vi "PI_GCS2_All_VIs.vi"   [LabVIEW 2020]
doc: "This VI contains all high level and low level VIs valid for PI GCS2 devices. \nSee diagram for a survey of all PI GCS2 high level and low level VIs. \nMenu / Browse / Show VI Hierarchy will show the file paths of the VIs. \nGlobal Variables are shown as Control as well as Indicator."
uses:
  Low Level/Communication.llb/Global1.vi
  Low Level/General command.llb/Controller names.ctl
  Low Level/Support.llb/Unbunde/bundle interface clusters for PI Terminal.vi
  Low Level/Communication.llb/Available DLL interfaces.ctl
  Low Level/Communication.llb/Available DLLs.ctl
  Low Level/Communication.llb/Available interfaces.ctl
  Low Level/Communication.llb/Termination character.ctl
  Low Level/General command.llb/Global2 (Array).vi
  Low Level/Communication.llb/Global DaisyChain.vi
  Low Level/Support.llb/HasCommandArray_Query.vi
  Low Level/Support.llb/GCSArray_regex_selector.ctl
  Low Level/Communication.llb/Syntax.ctl
  Low Level/General command.llb/CommandInfo.ctl
  Low Level/General command.llb/MemoryType.ctl
  Low Level/General command.llb/Parameter Set.ctl
  Low Level/General command.llb/ParameterInfoSet.ctl
  Low Level/General command.llb/UnitDescription.ctl
  Low Level/Special command.llb/UserCommandLevel.ctl
  Low Level/Communication.llb/Configuration Setup State.ctl
  Low Level/General command.llb/HardwareInfo.ctl
  Low Level/General command.llb/DynamicHardwareInfo.ctl
  Low Level/General command.llb/FirmwareInfo.ctl
  Low Level/Special command.llb/RecorderStatus.ctl
  Low Level/Special command.llb/RecorderTraceConfiguration.ctl
  Low Level/Special command.llb/RecorderTriggerConfiguration.ctl
  Low Level/Special command.llb/DriveStateMachine.ctl
  Low Level/Special command.llb/ModeOfOperation.ctl
  Low Level/General command.llb/AxisStatus.ctl
  Low Level/General command.llb/SystemStatus.ctl
  Low Level/General command.llb/Status.ctl
panel:
  # "PI GCS2 LabVIEW driver set"
  # "This VI contains all high level and low level VIs valid for PI GCS2 devices. See diagram for a survey of all PI GCS2 high level and low level VIs. Menu / Browse / Show VI Hierarchy will show the file paths of the VIs. Global Variables are shown as Control as well as Indicator."
types:
  T1 = typedef "Status.ctl" = cluster{"Element":string, "Status bits":bool[]}
  T2 = typedef "SystemStatus.ctl" = cluster{"Element":string, "Command Error":bool, "Critical Error":bool, "Information":bool, "Warning":bool}
  T3 = typedef "AxisStatus.ctl" = cluster{"Element":string, "Error":bool, "EAX?":bool, "Drive State Machine":T4, "Mode of Operation":T5, "OL/CL control active?":bool, "ONT?":bool, "In Motion":bool, "FRF?":bool, "IPR":bool, "Plim":bool, "Nlim":bool}
  T4 = typedef "DriveStateMachine.ctl" = u16
  T5 = typedef "ModeOfOperation.ctl" = enum16{"Open", "Open-Loop Position", "Closed-Loop Position", "Open-Loop Velocity", "Closed-Loop Velocity", "Open-Loop Force", "Closed-Loop Force", "Step Operation"}
  T6 = typedef "RecorderTriggerConfiguration.ctl" = cluster{"RecorderID":string, "RecorderTrigger":string, "AxisID":string, "Recurring":string}
  T7 = typedef "RecorderTraceConfiguration.ctl" = cluster{"RecorderID":string, "TraceID":i32, "Container Unit":string, "Function Unit":string, "ParameterID":i32}
  T8 = typedef "RecorderStatus.ctl" = enum16{"RUN", "CFG", "WAIT"}
  T9 = typedef "FirmwareInfo.ctl" = cluster{"Container Unit":string, "Function Unit":string, "ID":string, "Mathccode":string, "Version":string, "Date":string, "Compatibility":string, "Description":string}
  T10 = typedef "DynamicHardwareInfo.ctl" = cluster{"Property":string, "Type":string, "Value":string}
  T11 = typedef "HardwareInfo.ctl" = cluster{"Matchcode":string, "Version":string, "Serial Number":string, "Date":string, "Dynamic Hardware":cluster{"Property":string, "Type":string, "Value":string}[], "Firmware":cluster{"Container Unit":string, "Function Unit":string, "ID":string, "Mathccode":string, "Version":string, "Date":string, "Compatibility":string, "Description":string}[]}
  T12 = typedef "Configuration Setup State.ctl" = enum16{"Do nothing", "Initialize indicators", "Select Connection", "TCP/IP Connection", "RS232 Connection", "USB Connection", "Board Connection", "DaisyChain Connection", "Open Interface", "Read IDs", "Prepare referencing", "Reference", "Servo", "Query Status", "Misc", "WaveGenerator", "Control Mode", "Enable Axes", "Translate Error", "Hexapod", "Piezo"}
  T13 = typedef "UserCommandLevel.ctl" = enum16{"User", "Expert", "PI Staff", "FW Developer"}
  T14 = typedef "UnitDescription.ctl" = cluster{"Container Unit":string, "Function Unit":string, "Description":string}
  T15 = typedef "ParameterInfoSet.ctl" = cluster{"Container Unit":string, "Function Unit":string, "Parameter ID":string, "DataType":string, "Dimension":string, "Read UCL":string, "Write UCL":string, "Min Value":string, "Max Value":string, "Parameter Type":string, "Description":string}
  T16 = typedef "Parameter Set.ctl" = cluster{"Memory Type":T17, "Container Unit":string, "Function Unit":string, "Parameter ID":string, "Parameter Value":string}
  T17 = typedef "MemoryType.ctl" = enum16{"<No Setting>", "RAM", "FLASH", "TMP"}
  T18 = typedef "CommandInfo.ctl" = cluster{"Command":string, "Command Signatur":string, "Description":string}
  T19 = typedef "GCSArray_regex_selector.ctl" = enum16{"GCS_ARRAY Block Full", "GCS_ARRAY Block ID", "GCS_ARRAY Block Header", "GCS_ARRAY Block Data", "GCS_ARRAY Identifier", "GCS_ARRAY Remark", "GCS_ARRAY Version", "GCS_ARRAY Dimension", "GCS_ARRAY Type", "GCS_ARRAY Separator", "GCS_ARRAY NData", "GCS_ARRAY NData%", "GCS_ARRAY NData% Keyword", "GCS_ARRAY Name%", "GCS_ARRAY Name% Keyword", "GCS_ARRAY Start%", "GCS_ARRAY Start% Keyword", "GCS_ARRAY End%", "GCS_ARRAY End% Keyword", "GCS_ARRAY Delta%", "GCS_ARRAY Delta% Keword", "GCS_ARRAY Sample Time", "GCS_ARRAY Unit of transmitted value%", "GCS_ARRAY Trans_Unit% Keyword", "GCS_ARRAY Trans_Unit% = RAW Keyword", "GCS_ARRAY Unit of displayed value%", "GCS_ARRAY Disp_Unit% Keyword", "GCS_ARRAY Nominator%", "GCS_ARRAY Ratio_Nom% Keyword", "GCS_ARRAY Denominator%", "GCS_ARRAY Ratio_Denom% Keyword", "GCS_ARRAY End of Header", "GCS_ARRAY Empty line of Header"}
  T20 = typedef "Syntax.ctl" = enum16{"GCS 1.0", "GCS 2.0", "GCS 3.0"}
  T21 = typedef "Termination character.ctl" = enum16{"LF", "CR", "LFCR", "CRLF"}
  T22 = typedef "Available interfaces.ctl" = u16
  T23 = typedef "Available DLLs.ctl" = u16
  T24 = typedef "Available DLL interfaces.ctl" = u16
  T25 = typedef "Controller names.ctl" = enum16{"None", "Analog", "C-702", "C-413", "C-414", "C-843", "C-843.PM", "C-844", "C-848", "C-865", "C-866", "C-867", "C-877", "C-880", "C-884", "C-885", "C-886", "C-887", "C-891", "E-135", "E-516", "E-517", "E-518", "E-709", "E-710", "E-712", "E-725", "E-727", "E-753", "E-754", "E-755", "E-761", "E-816", "E-861", "E-870", "E-871", "E-872", "E-873", "E-874", "F-206", "HydraPollux", "M-840", "M-850", "M-8X0", "Mercury", "Mercury_GCS", "PI_GCS2"}
  T26 = cluster{"No. of devices":i32, "Port ID":i32, "Devices":string[], "Description":string}[]
  T27 = cluster{"Conn. axes":string[], "Controller name":T25}[]
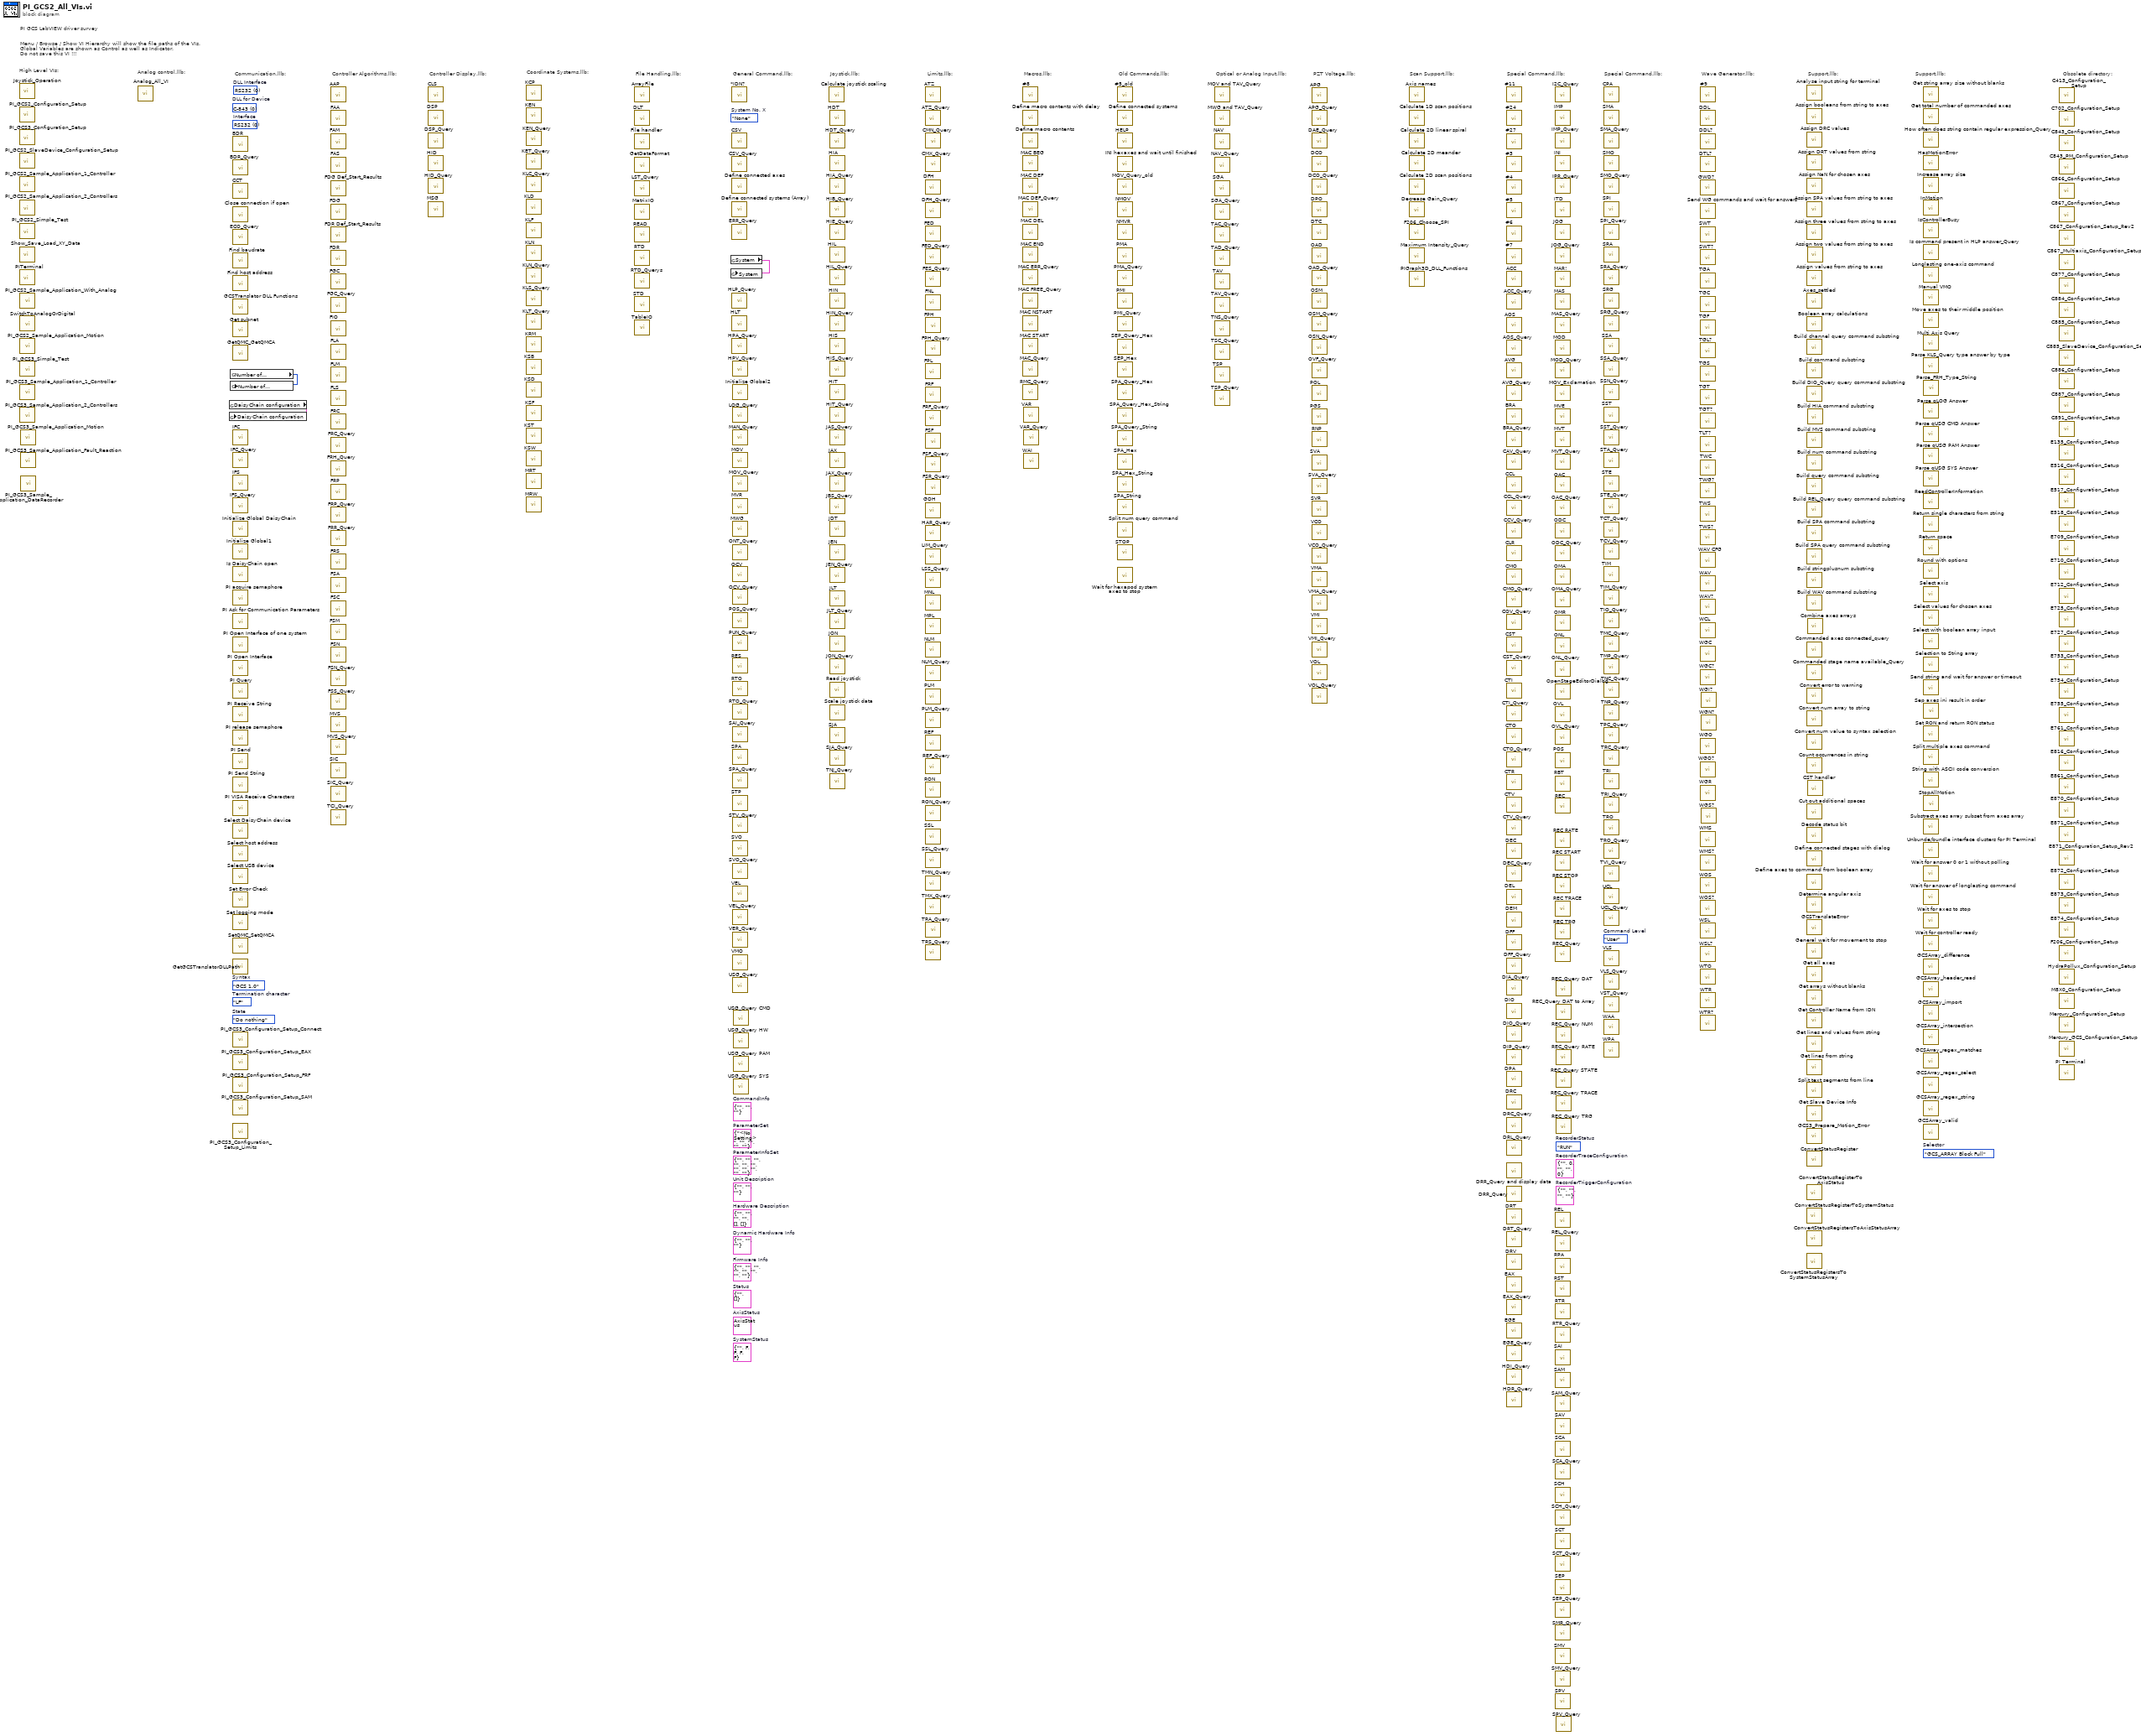
[diagram p0: block diagram]
diagram:
  (unwired) T1 {"Element"="", "Status bits"=[]}  # Status
  (unwired) T2 {"Element"="", "Command Error"=FALSE, "Critical Error"=FALSE, "Information"=FALSE, "Warning"=FALSE}  # SystemStatus
  (unwired) T3 {"Element"="", "Error"=FALSE, "EAX?"=FALSE, "Drive State Machine"=0, "Mode of Operation"=enum."Open", "OL/CL control active?"=FALSE, "ONT?"=FALSE, "In Motion"=FALSE, "FRF?"=FALSE, "IPR"=FALSE, "Plim"=FALSE, "Nlim"=FALSE}  # AxisStatus
  (unwired) T6 {"RecorderID"="", "RecorderTrigger"="", "AxisID"="", "Recurring"=""}  # RecorderTriggerConfiguration
  (unwired) T7 {"RecorderID"="", "TraceID"=0, "Container Unit"="", "Function Unit"="", "ParameterID"=0}  # RecorderTraceConfiguration
  (unwired) RecorderStatus."RUN"  # RecorderStatus
  (unwired) T9 {"Container Unit"="", "Function Unit"="", "ID"="", "Mathccode"="", "Version"="", "Date"="", "Compatibility"="", "Description"=""}  # Firmware Info
  (unwired) T10 {"Property"="", "Type"="", "Value"=""}  # Dynamic Hardware Info
  (unwired) T11 {"Matchcode"="", "Version"="", "Serial Number"="", "Date"="", "Dynamic Hardware"=[], "Firmware"=[]}  # Hardware Description
  (unwired) Configuration_Setup_State."Do nothing"  # State
  (unwired) UserCommandLevel."User"  # Command Level
  (unwired) T14 {"Container Unit"="", "Function Unit"="", "Description"=""}  # Unit Description
  (unwired) T15 {"Container Unit"="", "Function Unit"="", "Parameter ID"="", "DataType"="", "Dimension"="", "Read UCL"="", "Write UCL"="", "Min Value"="", "Max Value"="", "Parameter Type"="", "Description"=""}  # ParameterInfoSet
  (unwired) T16 {"Memory Type"=enum."<No Setting>", "Container Unit"="", "Function Unit"="", "Parameter ID"="", "Parameter Value"=""}  # ParameterSet
  (unwired) T18 {"Command"="", "Command Signatur"="", "Description"=""}  # CommandInfo
  (unwired) GCSArray_regex_selector."GCS_ARRAY Block Full"  # Selector
  (unwired) Syntax."GCS 1.0"  # Syntax
  (unwired) Termination_character."LF"  # Termination character
  (unwired) T22 0 items=["RS232", "GPIB", "DLL", "TCP-IP"]  # Interface
  (unwired) T23 0 items=["C-843", "C-844", "E-710", "C-843.PM", "C-865", "E-761", "Mercury", "E-755", "E-753", "C-866", "E-712", "E-725", "E-861", "C-867", "E-517", "E-816", "E-709", "PI_GCS2_DLL"]  # DLL for Device
  (unwired) T24 0 items=["RS232", "GPIB", "Board", "TCP-IP", "USB", "RS232_DC", "USB_DC"]  # DLL Interface
  (unwired) Controller_names."None"  # System No. X
  # "Obsolete directory:"
  # "Coordinate Systems.llb:"
  # "High Level VIs:"
  # "Analog control.llb:"
  # "Support.llb:"
  # "Wave Generator.llb:"
  # "Special Command.llb:"
  # "Support.llb:"
  # "Special Command.llb:"
  # "Scan Support.llb:"
  # "PZT Voltage.llb:"
  # "Optical or Analog Input.llb:"
  # "Old Commands.llb:"
  # "Macros.llb:"
  # "Limits.llb:"
  # "Joystick.llb:"
  # "General Command.llb:"
  # "File Handling.llb:"
  # "Controller Display.llb:"
  # "Controller Algorithms.llb:"
  # "Menu / Browse / Show VI Hierarchy will show the file paths of the VIs. \nGlobal Variables are shown as Control as well as Indicator.\nDo not save this VI !!!"
  # "PI GCS LabVIEW driver survey"
  # "Communication.llb:"
  n1 = call "Joystick_Operation.vi"() -> ()  [unwired: 15 in, 5 out]
  n2 = call "PI_GCS2_Configuration_Setup.vi"() -> ()  [unwired: 8 in, 12 out]
  n3 = call "PI_GCS3_Configuration_Setup.vi"() -> ()  [unwired: 14 in, 6 out]
  n4 = call "PI_GCS2_SlaveDevice_Configuration_Setup.vi"() -> ()  [unwired: 6 in, 14 out]
  n5 = call "PI_GCS2_Sample_Application_1_Controller.vi"() -> ()  [unwired: 1 out]
  n6 = call "PI_GCS2_Sample_Application_2_Controllers.vi"() -> ()  [unwired: 1 out]
  n7 = call "PI_GCS2_Simple_Test.vi"() -> ()  [unwired: 20 out]
  n8 = call "Show_Save_Load_XY_Data.vi"() -> ()  [unwired: 7 in, 13 out]
  n9 = call "PITerminal.vi"() -> ()  [unwired: 2 in, 18 out]
  n10 = call "PI_GCS2_Sample_Application_With_Analog.vi"() -> ()  [unwired: 1 out]
  n11 = call "SwitchToAnalogOrDigital.vi"() -> ()  [unwired: 9 in, 11 out]
  n12 = call "PI_GCS2_Sample_Application_Motion.vi"() -> ()  [unwired: 1 in]
  n13 = call "PI_GCS3_Simple_Test.vi"() -> ()  [unwired: 20 in]
  n14 = call "PI_GCS3_Sample_Application_1_Controller.vi"() -> ()  [unwired: 1 in]
  n15 = call "PI_GCS3_Sample_Application_2_Controllers.vi"() -> ()  [unwired: 1 in]
  n16 = call "PI_GCS3_Sample_Application_Motion.vi"() -> ()  [unwired: 1 in]
  n17 = call "PI_GCS3_Sample_Application_Fault_Reaction.vi"() -> ()  [unwired: 20 in]
  n18 = call "PI_GCS3_Sample_Application_DataRecorder.vi"() -> ()  [unwired: 20 in]
  n19 = call "Analog_All_VI.vi"() -> ()  [unwired: 12 out]
  n20 = global read "Global DaisyChain.vi" "DaisyChain configuration"() -> (w1:T26)
  n21 = global write "Global DaisyChain.vi" "DaisyChain configuration"(w1) -> ()
  n22 = global read "Global1.vi" "Number of\nsystems"() -> (w3:i32)
  n23 = global write "Global1.vi" "Number of\nsystems"(w3) -> ()
  n24 = call "BDR.vi"() -> ()  [unwired: 4 in, 16 out]
  n25 = call "BDR_Query.vi"() -> ()  [unwired: 2 in, 18 out]
  n26 = call "CCT.vi"() -> ()  [unwired: 3 in, 17 out]
  n27 = call "Close connection if open.vi"() -> ()  [unwired: 3 in, 17 out]
  n28 = call "ECO_Query.vi"() -> ()  [unwired: 3 in, 17 out]
  n29 = call "Find baudrate.vi"() -> ()  [unwired: 10 in, 10 out]
  n30 = call "Find host address.vi"() -> ()  [unwired: 6 in, 14 out]
  n31 = call "GCSTranslator DLL Functions.vi"() -> ()  [unwired: 7 in, 13 out]
  n32 = call "Get subnet.vi"() -> ()  [unwired: 20 out]
  n33 = call "GetQMC_GetQMCA.vi"() -> ()  [unwired: 6 in, 14 out]
  n34 = call "IFC.vi"() -> ()  [unwired: 4 in, 16 out]
  n35 = call "IFC_Query.vi"() -> ()  [unwired: 4 in, 16 out]
  n36 = call "IFS.vi"() -> ()  [unwired: 5 in, 15 out]
  n37 = call "IFS_Query.vi"() -> ()  [unwired: 4 in, 16 out]
  n38 = call "Initialize Global DaisyChain.vi"() -> ()  [unwired: 2 in, 18 out]
  n39 = call "Initialize Global1.vi"() -> ()  [unwired: 2 in, 18 out]
  n40 = call "Is DaisyChain open.vi"() -> ()  [unwired: 2 in, 18 out]
  n41 = call "PI acquire semaphore.vi"() -> ()  [unwired: 2 in, 18 out]
  n42 = call "PI Ask for Communication Parameters.vi"() -> ()  [unwired: 20 out]
  n43 = call "PI Open Interface of one system.vi"() -> ()  [unwired: 12 in, 8 out]
  n44 = call "PI Open Interface.vi"() -> ()  [unwired: 12 in, 8 out]
  n45 = call "PI Query.vi"() -> ()  [unwired: 7 in, 13 out]
  n46 = call "PI Receive String.vi"() -> ()  [unwired: 3 in, 17 out]
  n47 = call "PI release semaphore.vi"() -> ()  [unwired: 4 in, 16 out]
  n48 = call "PI Send.vi"() -> ()  [unwired: 6 in, 14 out]
  n49 = call "PI Send String.vi"() -> ()  [unwired: 4 in, 16 out]
  n50 = call "PI VISA Receive Characters.vi"() -> ()  [unwired: 3 in, 17 out]
  n51 = call "Select DaisyChain device.vi"() -> ()  [unwired: 9 in, 11 out]
  n52 = call "Select host address.vi"() -> ()  [unwired: 6 in, 14 out]
  n53 = call "Select USB device.vi"() -> ()  [unwired: 5 in, 15 out]
  n54 = call "Set Error Check.vi"() -> ()  [unwired: 2 in, 10 out]
  n55 = call "Set logging mode.vi"() -> ()  [unwired: 4 in, 16 out]
  n56 = call "SetQMC_SetQMCA.vi"() -> ()  [unwired: 8 in, 12 out]
  n57 = call "GetGCSTranslatorDLLPath.vi"() -> ()  [unwired: 1 in, 1 out]
  n58 = call "PI_GCS3_Configuration_Setup_Connect.vi"() -> ()  [unwired: 19 in, 1 out]
  n59 = call "PI_GCS3_Configuration_Setup_EAX.vi"() -> ()  [unwired: 19 in, 1 out]
  n60 = call "PI_GCS3_Configuration_Setup_FRF.vi"() -> ()  [unwired: 19 in, 1 out]
  n61 = call "PI_GCS3_Configuration_Setup_SAM.vi"() -> ()  [unwired: 19 in, 1 out]
  n62 = call "PI_GCS3_Configuration_Setup_Limits.vi"() -> ()  [unwired: 17 in, 3 out]
  n63 = call "AAP.vi"() -> ()  [unwired: 12 in, 8 out]
  n64 = call "FAA.vi"() -> ()  [unwired: 11 in, 9 out]
  n65 = call "FAM.vi"() -> ()  [unwired: 11 in, 9 out]
  n66 = call "FAS.vi"() -> ()  [unwired: 11 in, 9 out]
  n67 = call "FDG Def_Start_Results.vi"() -> ()  [unwired: 12 in, 8 out]
  n68 = call "FDG.vi"() -> ()  [unwired: 12 in, 8 out]
  n69 = call "FDR Def_Start_Results.vi"() -> ()  [unwired: 12 in, 8 out]
  n70 = call "FDR.vi"() -> ()  [unwired: 14 in, 6 out]
  n71 = call "FGC.vi"() -> ()  [unwired: 7 in, 13 out]
  n72 = call "FGC_Query.vi"() -> ()  [unwired: 4 in, 16 out]
  n73 = call "FIO.vi"() -> ()  [unwired: 13 in, 7 out]
  n74 = call "FLA.vi"() -> ()  [unwired: 13 in, 7 out]
  n75 = call "FLM.vi"() -> ()  [unwired: 13 in, 7 out]
  n76 = call "FLS.vi"() -> ()  [unwired: 13 in, 7 out]
  n77 = call "FRC.vi"() -> ()  [unwired: 5 in, 15 out]
  n78 = call "FRC_Query.vi"() -> ()  [unwired: 4 in, 16 out]
  n79 = call "FRH_Query.vi"() -> ()  [unwired: 2 in, 18 out]
  n80 = call "FRP.vi"() -> ()  [unwired: 4 in, 16 out]
  n81 = call "FRP_Query.vi"() -> ()  [unwired: 4 in, 16 out]
  n82 = call "FRR_Query.vi"() -> ()  [unwired: 6 in, 14 out]
  n83 = call "FRS.vi"() -> ()  [unwired: 3 in, 17 out]
  n84 = call "FSA.vi"() -> ()  [unwired: 13 in, 7 out]
  n85 = call "FSC.vi"() -> ()  [unwired: 12 in, 8 out]
  n86 = call "FSM.vi"() -> ()  [unwired: 12 in, 8 out]
  n87 = call "FSN.vi"() -> ()  [unwired: 13 in, 7 out]
  n88 = call "FSN_Query.vi"() -> ()  [unwired: 3 in, 17 out]
  n89 = call "FSS_Query.vi"() -> ()  [unwired: 2 in, 18 out]
  n90 = call "MVS.vi"() -> ()  [unwired: 8 in, 12 out]
  n91 = call "MVS_Query.vi"() -> ()  [unwired: 5 in, 15 out]
  n92 = call "SIC.vi"() -> ()  [unwired: 6 in, 14 out]
  n93 = call "SIC_Query.vi"() -> ()  [unwired: 4 in, 16 out]
  n94 = call "TCI_Query.vi"() -> ()  [unwired: 3 in, 17 out]
  n95 = call "CLS.vi"() -> ()  [unwired: 2 in, 18 out]
  n96 = call "DSP.vi"() -> ()  [unwired: 5 in, 15 out]
  n97 = call "DSP_Query.vi"() -> ()  [unwired: 3 in, 17 out]
  n98 = call "HID.vi"() -> ()  [unwired: 5 in, 15 out]
  n99 = call "HID_Query.vi"() -> ()  [unwired: 3 in, 17 out]
  n100 = call "MSG.vi"() -> ()  [unwired: 3 in, 17 out]
  n101 = call "KCP.vi"() -> ()  [unwired: 4 in, 16 out]
  n102 = call "KEN.vi"() -> ()  [unwired: 3 in, 17 out]
  n103 = call "KEN_Query.vi"() -> ()  [unwired: 3 in, 17 out]
  n104 = call "KET_Query.vi"() -> ()  [unwired: 3 in, 17 out]
  n105 = call "KLC_Query.vi"() -> ()  [unwired: 6 in, 14 out]
  n106 = call "KLD.vi"() -> ()  [unwired: 6 in, 14 out]
  n107 = call "KLF.vi"() -> ()  [unwired: 3 in, 17 out]
  n108 = call "KLN.vi"() -> ()  [unwired: 4 in, 16 out]
  n109 = call "KLN_Query.vi"() -> ()  [unwired: 3 in, 17 out]
  n110 = call "KLS_Query.vi"() -> ()  [unwired: 5 in, 15 out]
  n111 = call "KLT_Query.vi"() -> ()  [unwired: 4 in, 16 out]
  n112 = call "KRM.vi"() -> ()  [unwired: 3 in, 17 out]
  n113 = call "KSB.vi"() -> ()  [unwired: 6 in, 14 out]
  n114 = call "KSD.vi"() -> ()  [unwired: 6 in, 14 out]
  n115 = call "KSF.vi"() -> ()  [unwired: 3 in, 17 out]
  n116 = call "KST.vi"() -> ()  [unwired: 6 in, 14 out]
  n117 = call "KSW.vi"() -> ()  [unwired: 6 in, 14 out]
  n118 = call "MRT.vi"() -> ()  [unwired: 5 in, 15 out]
  n119 = call "MRW.vi"() -> ()  [unwired: 5 in, 15 out]
  n120 = call "ArrayFile.vi"() -> ()  [unwired: 20 out]
  n121 = call "DLT.vi"() -> ()  [unwired: 3 in, 17 out]
  n122 = call "File handler.vi"() -> ()  [unwired: 6 in, 14 out]
  n123 = call "GetDataFormat.vi"() -> ()  [unwired: 2 in, 18 out]
  n124 = call "LST_Query.vi"() -> ()  [unwired: 2 in, 18 out]
  n125 = call "MatrixIO.vi"() -> ()  [unwired: 7 in, 13 out]
  n126 = call "READ.vi"() -> ()  [unwired: 3 in, 17 out]
  n127 = call "RTD.vi"() -> ()  [unwired: 5 in, 15 out]
  n128 = call "RTD_Querys.vi"() -> ()  [unwired: 2 in, 18 out]
  n129 = call "STD.vi"() -> ()  [unwired: 5 in, 15 out]
  n130 = call "TableIO.vi"() -> ()  [unwired: 6 in, 14 out]
  n131 = global read "Global2 (Array).vi" "System"() -> (w2:T27)
  n132 = global write "Global2 (Array).vi" "System"(w2) -> ()
  n133 = call "*IDN?.vi"() -> ()  [unwired: 2 in, 18 out]
  n134 = call "CSV.vi"() -> ()  [unwired: 3 in, 17 out]
  n135 = call "CSV_Query.vi"() -> ()  [unwired: 2 in, 18 out]
  n136 = call "Define connected axes.vi"() -> ()  [unwired: 5 in, 15 out]
  n137 = call "Define connected systems (Array).vi"() -> ()  [unwired: 4 in, 16 out]
  n138 = call "ERR_Query.vi"() -> ()  [unwired: 2 in, 18 out]
  n139 = call "HLP_Query.vi"() -> ()  [unwired: 2 in, 18 out]
  n140 = call "HLT.vi"() -> ()  [unwired: 5 in, 15 out]
  n141 = call "HPA_Query.vi"() -> ()  [unwired: 2 in, 18 out]
  n142 = call "HPV_Query.vi"() -> ()  [unwired: 2 in, 18 out]
  n143 = call "Initialize Global2.vi"() -> ()  [unwired: 2 in, 18 out]
  n144 = call "LOG_Query.vi"() -> ()  [unwired: 18 in, 2 out]
  n145 = call "MAN_Query.vi"() -> ()  [unwired: 3 in, 17 out]
  n146 = call "MOV.vi"() -> ()  [unwired: 5 in, 15 out]
  n147 = call "MOV_Query.vi"() -> ()  [unwired: 5 in, 15 out]
  n148 = call "MVR.vi"() -> ()  [unwired: 5 in, 15 out]
  n149 = call "MWG.vi"() -> ()  [unwired: 5 in, 15 out]
  n150 = call "ONT_Query.vi"() -> ()  [unwired: 5 in, 15 out]
  n151 = call "OCV.vi"() -> ()  [unwired: 19 in, 1 out]
  n152 = call "OCV_Query.vi"() -> ()  [unwired: 18 in, 2 out]
  n153 = call "POS_Query.vi"() -> ()  [unwired: 5 in, 15 out]
  n154 = call "PUN_Query.vi"() -> ()  [unwired: 5 in, 15 out]
  n155 = call "RES.vi"() -> ()  [unwired: 19 in, 1 out]
  n156 = call "RTO.vi"() -> ()  [unwired: 5 in, 15 out]
  n157 = call "RTO_Query.vi"() -> ()  [unwired: 5 in, 15 out]
  n158 = call "SAI_Query.vi"() -> ()  [unwired: 5 in, 15 out]
  n159 = call "SPA.vi"() -> ()  [unwired: 10 in, 10 out]
  n160 = call "SPA_Query.vi"() -> ()  [unwired: 7 in, 13 out]
  n161 = call "STP.vi"() -> ()  [unwired: 2 in, 18 out]
  n162 = call "STV_Query.vi"() -> ()  [unwired: 18 in, 2 out]
  n163 = call "SVO.vi"() -> ()  [unwired: 5 in, 15 out]
  n164 = call "SVO_Query.vi"() -> ()  [unwired: 5 in, 15 out]
  n165 = call "VEL.vi"() -> ()  [unwired: 6 in, 14 out]
  n166 = call "VEL_Query.vi"() -> ()  [unwired: 5 in, 15 out]
  n167 = call "VER_Query.vi"() -> ()  [unwired: 2 in, 18 out]
  n168 = call "VMO.vi"() -> ()  [unwired: 5 in, 15 out]
  n169 = call-poly "USG_Query.vi"() -> ()  [unwired: 18 in, 2 out]
  n170 = call "USG_Query CMD.vi"() -> ()  [unwired: 18 in, 2 out]
  n171 = call "USG_Query HW.vi"() -> ()  [unwired: 18 in, 2 out]
  n172 = call "USG_Query PAM.vi"() -> ()  [unwired: 18 in, 2 out]
  n173 = call "USG_Query SYS.vi"() -> ()  [unwired: 18 in, 2 out]
  n174 = call "Calculate joystick scaling.vi"() -> ()  [unwired: 6 in, 14 out]
  n175 = call "HDT.vi"() -> ()  [unwired: 5 in, 15 out]
  n176 = call "HDT_Query.vi"() -> ()  [unwired: 5 in, 15 out]
  n177 = call "HIA.vi"() -> ()  [unwired: 6 in, 14 out]
  n178 = call "HIA_Query.vi"() -> ()  [unwired: 5 in, 15 out]
  n179 = call "HIB_Query.vi"() -> ()  [unwired: 5 in, 15 out]
  n180 = call "HIE_Query.vi"() -> ()  [unwired: 5 in, 15 out]
  n181 = call "HIL.vi"() -> ()  [unwired: 5 in, 15 out]
  n182 = call "HIL_Query.vi"() -> ()  [unwired: 5 in, 15 out]
  n183 = call "HIN.vi"() -> ()  [unwired: 4 in, 16 out]
  n184 = call "HIN_Query.vi"() -> ()  [unwired: 5 in, 15 out]
  n185 = call "HIS.vi"() -> ()  [unwired: 6 in, 14 out]
  n186 = call "HIS_Query.vi"() -> ()  [unwired: 6 in, 14 out]
  n187 = call "HIT.vi"() -> ()  [unwired: 5 in, 15 out]
  n188 = call "HIT_Query.vi"() -> ()  [unwired: 7 in, 13 out]
  n189 = call "JAS_Query.vi"() -> ()  [unwired: 5 in, 15 out]
  n190 = call "JAX.vi"() -> ()  [unwired: 5 in, 15 out]
  n191 = call "JAX_Query.vi"() -> ()  [unwired: 5 in, 15 out]
  n192 = call "JBS_Query.vi"() -> ()  [unwired: 5 in, 15 out]
  n193 = call "JDT.vi"() -> ()  [unwired: 5 in, 15 out]
  n194 = call "JEN.vi"() -> ()  [unwired: 3 in, 17 out]
  n195 = call "JEN_Query.vi"() -> ()  [unwired: 2 in, 18 out]
  n196 = call "JLT.vi"() -> ()  [unwired: 7 in, 13 out]
  n197 = call "JLT_Query.vi"() -> ()  [unwired: 7 in, 13 out]
  n198 = call "JON.vi"() -> ()  [unwired: 4 in, 16 out]
  n199 = call "JON_Query.vi"() -> ()  [unwired: 4 in, 16 out]
  n200 = call "Read joystick.vi"() -> ()  [unwired: 2 in, 18 out]
  n201 = call "Scale joystick data.vi"() -> ()  [unwired: 8 in, 12 out]
  n202 = call "SJA.vi"() -> ()  [unwired: 4 in, 16 out]
  n203 = call "SJA_Query.vi"() -> ()  [unwired: 3 in, 17 out]
  n204 = call "TNJ_Query.vi"() -> ()  [unwired: 2 in, 18 out]
  n205 = call "ATZ.vi"() -> ()  [unwired: 6 in, 14 out]
  n206 = call "ATZ_Query.vi"() -> ()  [unwired: 5 in, 15 out]
  n207 = call "DFH.vi"() -> ()  [unwired: 5 in, 15 out]
  n208 = call "DFH_Query.vi"() -> ()  [unwired: 5 in, 15 out]
  n209 = call "FED.vi"() -> ()  [unwired: 5 in, 15 out]
  n210 = call "FED_Query.vi"() -> ()  [unwired: 5 in, 15 out]
  n211 = call "FES_Query.vi"() -> ()  [unwired: 5 in, 15 out]
  n212 = call "FNL.vi"() -> ()  [unwired: 5 in, 15 out]
  n213 = call "FPL.vi"() -> ()  [unwired: 5 in, 15 out]
  n214 = call "FRF.vi"() -> ()  [unwired: 5 in, 15 out]
  n215 = call "FRF_Query.vi"() -> ()  [unwired: 5 in, 15 out]
  n216 = call "GOH.vi"() -> ()  [unwired: 5 in, 15 out]
  n217 = call "HAR_Query.vi"() -> ()  [unwired: 5 in, 15 out]
  n218 = call "LIM_Query.vi"() -> ()  [unwired: 5 in, 15 out]
  n219 = call "LSS_Query.vi"() -> ()  [unwired: 5 in, 15 out]
  n220 = call "MNL.vi"() -> ()  [unwired: 5 in, 15 out]
  n221 = call "MPL.vi"() -> ()  [unwired: 5 in, 15 out]
  n222 = call "NLM.vi"() -> ()  [unwired: 5 in, 15 out]
  n223 = call "NLM_Query.vi"() -> ()  [unwired: 5 in, 15 out]
  n224 = call "PLM.vi"() -> ()  [unwired: 5 in, 15 out]
  n225 = call "PLM_Query.vi"() -> ()  [unwired: 5 in, 15 out]
  n226 = call "REF.vi"() -> ()  [unwired: 5 in, 15 out]
  n227 = call "REF_Query.vi"() -> ()  [unwired: 5 in, 15 out]
  n228 = call "RON.vi"() -> ()  [unwired: 5 in, 15 out]
  n229 = call "RON_Query.vi"() -> ()  [unwired: 5 in, 15 out]
  n230 = call "SSL.vi"() -> ()  [unwired: 5 in, 15 out]
  n231 = call "SSL_Query.vi"() -> ()  [unwired: 5 in, 15 out]
  n232 = call "TMN_Query.vi"() -> ()  [unwired: 5 in, 15 out]
  n233 = call "TMX_Query.vi"() -> ()  [unwired: 5 in, 15 out]
  n234 = call "TRS_Query.vi"() -> ()  [unwired: 5 in, 15 out]
  n235 = call "CMN_Query.vi"() -> ()  [unwired: 5 in, 15 out]
  n236 = call "CMX_Query.vi"() -> ()  [unwired: 5 in, 15 out]
  n237 = call "FPH.vi"() -> ()  [unwired: 5 in, 15 out]
  n238 = call "FPH_Query.vi"() -> ()  [unwired: 5 in, 15 out]
  n239 = call "FSF.vi"() -> ()  [unwired: 8 in, 12 out]
  n240 = call "FSF_Query.vi"() -> ()  [unwired: 5 in, 15 out]
  n241 = call "FSR_Query.vi"() -> ()  [unwired: 4 in, 16 out]
  n242 = call "TRA_Query.vi"() -> ()  [unwired: 5 in, 15 out]
  n243 = call "#8.vi"() -> ()  [unwired: 2 in, 18 out]
  n244 = call "Define macro contents with delay.vi"() -> ()  [unwired: 4 in, 16 out]
  n245 = call "Define macro contents.vi"() -> ()  [unwired: 3 in, 17 out]
  n246 = call "MAC BEG.vi"() -> ()  [unwired: 3 in, 17 out]
  n247 = call "MAC DEF.vi"() -> ()  [unwired: 3 in, 17 out]
  n248 = call "MAC DEF_Query.vi"() -> ()  [unwired: 2 in, 18 out]
  n249 = call "MAC DEL.vi"() -> ()  [unwired: 4 in, 16 out]
  n250 = call "MAC END.vi"() -> ()  [unwired: 2 in, 18 out]
  n251 = call "MAC ERR_Query.vi"() -> ()  [unwired: 2 in, 18 out]
  n252 = call "MAC FREE_Query.vi"() -> ()  [unwired: 2 in, 18 out]
  n253 = call "MAC NSTART.vi"() -> ()  [unwired: 5 in, 15 out]
  n254 = call "MAC START.vi"() -> ()  [unwired: 4 in, 16 out]
  n255 = call "MAC_Query.vi"() -> ()  [unwired: 4 in, 16 out]
  n256 = call "RMC_Query.vi"() -> ()  [unwired: 2 in, 18 out]
  n257 = call "VAR.vi"() -> ()  [unwired: 4 in, 16 out]
  n258 = call "VAR_Query.vi"() -> ()  [unwired: 4 in, 16 out]
  n259 = call "WAI.vi"() -> ()  [unwired: 5 in, 15 out]
  n260 = call "#5_old.vi"() -> ()  [unwired: 2 in, 18 out]
  n261 = call "Define connected systems.vi"() -> ()  [unwired: 4 in, 16 out]
  n262 = call "HELP.vi"() -> ()  [unwired: 2 in, 18 out]
  n263 = call "INI hexaxes and wait until finished.vi"() -> ()  [unwired: 6 in, 14 out]
  n264 = call "MOV_Query_old.vi"() -> ()  [unwired: 3 in, 17 out]
  n265 = call "NMOV.vi"() -> ()  [unwired: 5 in, 15 out]
  n266 = call "NMVR.vi"() -> ()  [unwired: 5 in, 15 out]
  n267 = call "PMA.vi"() -> ()  [unwired: 5 in, 15 out]
  n268 = call "PMA_Query.vi"() -> ()  [unwired: 5 in, 15 out]
  n269 = call "PMI.vi"() -> ()  [unwired: 5 in, 15 out]
  n270 = call "PMI_Query.vi"() -> ()  [unwired: 5 in, 15 out]
  n271 = call "SEP_Query_Hex.vi"() -> ()  [unwired: 5 in, 15 out]
  n272 = call "SEP_Hex.vi"() -> ()  [unwired: 6 in, 14 out]
  n273 = call "SPA_Query_Hex.vi"() -> ()  [unwired: 5 in, 15 out]
  n274 = call "SPA_Query_Hex_String.vi"() -> ()  [unwired: 5 in, 15 out]
  n275 = call "SPA_Query_String.vi"() -> ()  [unwired: 4 in, 16 out]
  n276 = call "SPA_Hex.vi"() -> ()  [unwired: 6 in, 14 out]
  n277 = call "SPA_Hex_String.vi"() -> ()  [unwired: 5 in, 15 out]
  n278 = call "SPA_String.vi"() -> ()  [unwired: 5 in, 15 out]
  n279 = call "Split num query command.vi"() -> ()  [unwired: 4 in, 16 out]
  n280 = call "STOP.vi"() -> ()  [unwired: 2 in, 18 out]
  n281 = call "Wait for hexapod system axes to stop.vi"() -> ()  [unwired: 5 in, 15 out]
  n282 = call "MOV and TAV_Query.vi"() -> ()  [unwired: 9 in, 11 out]
  n283 = call "MWG and TAV_Query.vi"() -> ()  [unwired: 9 in, 11 out]
  n284 = call "NAV.vi"() -> ()  [unwired: 4 in, 16 out]
  n285 = call "NAV_Query.vi"() -> ()  [unwired: 3 in, 17 out]
  n286 = call "SGA.vi"() -> ()  [unwired: 4 in, 16 out]
  n287 = call "SGA_Query.vi"() -> ()  [unwired: 3 in, 17 out]
  n288 = call "TAC_Query.vi"() -> ()  [unwired: 2 in, 18 out]
  n289 = call "TAD_Query.vi"() -> ()  [unwired: 5 in, 15 out]
  n290 = call "TAV.vi"() -> ()  [unwired: 7 in, 13 out]
  n291 = call "TAV_Query.vi"() -> ()  [unwired: 4 in, 16 out]
  n292 = call "TNS_Query.vi"() -> ()  [unwired: 5 in, 15 out]
  n293 = call "TSC_Query.vi"() -> ()  [unwired: 2 in, 18 out]
  n294 = call "TSP.vi"() -> ()  [unwired: 5 in, 15 out]
  n295 = call "TSP_Query.vi"() -> ()  [unwired: 5 in, 15 out]
  n296 = call "APG.vi"() -> ()  [unwired: 5 in, 15 out]
  n297 = call "APG_Query.vi"() -> ()  [unwired: 5 in, 15 out]
  n298 = call "DAE_Query.vi"() -> ()  [unwired: 5 in, 15 out]
  n299 = call "DCO.vi"() -> ()  [unwired: 4 in, 16 out]
  n300 = call "DCO_Query.vi"() -> ()  [unwired: 5 in, 15 out]
  n301 = call "DPO.vi"() -> ()  [unwired: 5 in, 15 out]
  n302 = call "DTC.vi"() -> ()  [unwired: 4 in, 16 out]
  n303 = call "OAD.vi"() -> ()  [unwired: 5 in, 15 out]
  n304 = call "OAD_Query.vi"() -> ()  [unwired: 5 in, 15 out]
  n305 = call "OSM.vi"() -> ()  [unwired: 5 in, 15 out]
  n306 = call "OSM_Query.vi"() -> ()  [unwired: 5 in, 15 out]
  n307 = call "OSN_Query.vi"() -> ()  [unwired: 5 in, 15 out]
  n308 = call "OVF_Query.vi"() -> ()  [unwired: 5 in, 15 out]
  n309 = call "POL.vi"() -> ()  [unwired: 4 in, 16 out]
  n310 = call "PGS.vi"() -> ()  [unwired: 5 in, 15 out]
  n311 = call "RNP.vi"() -> ()  [unwired: 6 in, 14 out]
  n312 = call "SVA.vi"() -> ()  [unwired: 5 in, 15 out]
  n313 = call "SVA_Query.vi"() -> ()  [unwired: 5 in, 15 out]
  n314 = call "SVR.vi"() -> ()  [unwired: 5 in, 15 out]
  n315 = call "VCO.vi"() -> ()  [unwired: 4 in, 16 out]
  n316 = call "VCO_Query.vi"() -> ()  [unwired: 5 in, 15 out]
  n317 = call "VMA.vi"() -> ()  [unwired: 5 in, 15 out]
  n318 = call "VMA_Query.vi"() -> ()  [unwired: 5 in, 15 out]
  n319 = call "VMI.vi"() -> ()  [unwired: 5 in, 15 out]
  n320 = call "VMI_Query.vi"() -> ()  [unwired: 5 in, 15 out]
  n321 = call "VOL.vi"() -> ()  [unwired: 5 in, 15 out]
  n322 = call "VOL_Query.vi"() -> ()  [unwired: 5 in, 15 out]
  n323 = call "Axis names.vi"() -> ()  [unwired: 1 in, 19 out]
  n324 = call "Calculate 1D scan positions.vi"() -> ()  [unwired: 4 in, 16 out]
  n325 = call "Calculate 2D linear spiral.vi"() -> ()  [unwired: 4 in, 16 out]
  n326 = call "Calculate 2D meander.vi"() -> ()  [unwired: 8 in, 12 out]
  n327 = call "Calculate 2D scan positions.vi"() -> ()  [unwired: 7 in, 13 out]
  n328 = call "Decrease Gain_Query.vi"() -> ()  [unwired: 6 in, 14 out]
  n329 = call "F206_Choose_SPI.vi"() -> ()  [unwired: 4 in, 16 out]
  n330 = call "Maximum Intensity_Query.vi"() -> ()  [unwired: 8 in, 12 out]
  n331 = call "PIGraph3D_DLL_Functions.vi"() -> ()  [unwired: 13 in, 7 out]
  n332 = call "#11.vi"() -> ()  [unwired: 2 in, 18 out]
  n333 = call "#24.vi"() -> ()  [unwired: 2 in, 18 out]
  n334 = call "#27.vi"() -> ()  [unwired: 2 in, 18 out]
  n335 = call "#3.vi"() -> ()  [unwired: 2 in, 18 out]
  n336 = call "#4.vi"() -> ()  [unwired: 2 in, 18 out]
  n337 = call "#5.vi"() -> ()  [unwired: 2 in, 18 out]
  n338 = call "#6.vi"() -> ()  [unwired: 2 in, 18 out]
  n339 = call "#7.vi"() -> ()  [unwired: 2 in, 18 out]
  n340 = call "ACC.vi"() -> ()  [unwired: 6 in, 14 out]
  n341 = call "ACC_Query.vi"() -> ()  [unwired: 5 in, 15 out]
  n342 = call "AOS.vi"() -> ()  [unwired: 5 in, 15 out]
  n343 = call "AOS_Query.vi"() -> ()  [unwired: 5 in, 15 out]
  n344 = call "AVG.vi"() -> ()  [unwired: 3 in, 17 out]
  n345 = call "AVG_Query.vi"() -> ()  [unwired: 2 in, 18 out]
  n346 = call "BRA.vi"() -> ()  [unwired: 4 in, 16 out]
  n347 = call "BRA_Query.vi"() -> ()  [unwired: 5 in, 15 out]
  n348 = call "CAV_Query.vi"() -> ()  [unwired: 5 in, 15 out]
  n349 = call "CCL.vi"() -> ()  [unwired: 4 in, 16 out]
  n350 = call "CLR.vi"() -> ()  [unwired: 5 in, 15 out]
  n351 = call "CMO_Query.vi"() -> ()  [unwired: 5 in, 15 out]
  n352 = call "COV_Query.vi"() -> ()  [unwired: 4 in, 16 out]
  n353 = call "CST.vi"() -> ()  [unwired: 4 in, 16 out]
  n354 = call "CST_Query.vi"() -> ()  [unwired: 5 in, 15 out]
  n355 = call "CTI.vi"() -> ()  [unwired: 6 in, 14 out]
  n356 = call "CTI_Query.vi"() -> ()  [unwired: 5 in, 15 out]
  n357 = call "CTO.vi"() -> ()  [unwired: 6 in, 14 out]
  n358 = call "CTO_Query.vi"() -> ()  [unwired: 5 in, 15 out]
  n359 = call "CTR.vi"() -> ()  [unwired: 5 in, 15 out]
  n360 = call "CTV.vi"() -> ()  [unwired: 5 in, 15 out]
  n361 = call "DEC.vi"() -> ()  [unwired: 6 in, 14 out]
  n362 = call "DEC_Query.vi"() -> ()  [unwired: 5 in, 15 out]
  n363 = call "DEL.vi"() -> ()  [unwired: 3 in, 17 out]
  n364 = call "DEM.vi"() -> ()  [unwired: 2 in, 18 out]
  n365 = call "DFF.vi"() -> ()  [unwired: 5 in, 15 out]
  n366 = call "DFF_Query.vi"() -> ()  [unwired: 5 in, 15 out]
  n367 = call "DIA_Query.vi"() -> ()  [unwired: 4 in, 16 out]
  n368 = call "DIO.vi"() -> ()  [unwired: 6 in, 14 out]
  n369 = call "DIO_Query.vi"() -> ()  [unwired: 6 in, 14 out]
  n370 = call "DIP_Query.vi"() -> ()  [unwired: 5 in, 15 out]
  n371 = call "DPA.vi"() -> ()  [unwired: 7 in, 13 out]
  n372 = call "DRC.vi"() -> ()  [unwired: 6 in, 14 out]
  n373 = call "DRC_Query.vi"() -> ()  [unwired: 4 in, 16 out]
  n374 = call "DRL_Query.vi"() -> ()  [unwired: 4 in, 16 out]
  n375 = call "DRR_Query and display data.vi"() -> ()  [unwired: 7 in, 13 out]
  n376 = call "DRR_Query.vi"() -> ()  [unwired: 8 in, 12 out]
  n377 = call "DRT.vi"() -> ()  [unwired: 5 in, 15 out]
  n378 = call "DRT_Query.vi"() -> ()  [unwired: 4 in, 16 out]
  n379 = call "DRV.vi"() -> ()  [unwired: 4 in, 16 out]
  n380 = call "EAX.vi"() -> ()  [unwired: 4 in, 16 out]
  n381 = call "EGE.vi"() -> ()  [unwired: 5 in, 15 out]
  n382 = call "EGE_Query.vi"() -> ()  [unwired: 5 in, 15 out]
  n383 = call "HDI_Query.vi"() -> ()  [unwired: 2 in, 18 out]
  n384 = call "HDR_Query.vi"() -> ()  [unwired: 3 in, 17 out]
  n385 = call "CCL_Query.vi"() -> ()  [unwired: 2 in, 18 out]
  n386 = call "CCV_Query.vi"() -> ()  [unwired: 5 in, 15 out]
  n387 = call "CMO.vi"() -> ()  [unwired: 4 in, 16 out]
  n388 = call "CTV_Query.vi"() -> ()  [unwired: 5 in, 15 out]
  n389 = call "EAX_Query.vi"() -> ()  [unwired: 5 in, 15 out]
  n390 = call "I2C_Query.vi"() -> ()  [unwired: 2 in, 18 out]
  n391 = call "IMP.vi"() -> ()  [unwired: 5 in, 15 out]
  n392 = call "IMP_Query.vi"() -> ()  [unwired: 6 in, 14 out]
  n393 = call "INI.vi"() -> ()  [unwired: 5 in, 15 out]
  n394 = call "IPR_Query.vi"() -> ()  [unwired: 18 in, 2 out]
  n395 = call "ITD.vi"() -> ()  [unwired: 5 in, 15 out]
  n396 = call "JOG.vi"() -> ()  [unwired: 5 in, 15 out]
  n397 = call "JOG_Query.vi"() -> ()  [unwired: 5 in, 15 out]
  n398 = call "MAR!.vi"() -> ()  [unwired: 5 in, 15 out]
  n399 = call "MAS.vi"() -> ()  [unwired: 4 in, 16 out]
  n400 = call "MAS_Query.vi"() -> ()  [unwired: 5 in, 15 out]
  n401 = call "MOV_Exclamation.vi"() -> ()  [unwired: 5 in, 15 out]
  n402 = call "MVE.vi"() -> ()  [unwired: 5 in, 15 out]
  n403 = call "MVT.vi"() -> ()  [unwired: 5 in, 15 out]
  n404 = call "MVT_Query.vi"() -> ()  [unwired: 5 in, 15 out]
  n405 = call "OAC.vi"() -> ()  [unwired: 6 in, 14 out]
  n406 = call "OAC_Query.vi"() -> ()  [unwired: 5 in, 15 out]
  n407 = call "ODC.vi"() -> ()  [unwired: 6 in, 14 out]
  n408 = call "ODC_Query.vi"() -> ()  [unwired: 5 in, 15 out]
  n409 = call "OMA.vi"() -> ()  [unwired: 5 in, 15 out]
  n410 = call "OMA_Query.vi"() -> ()  [unwired: 5 in, 15 out]
  n411 = call "OMR.vi"() -> ()  [unwired: 5 in, 15 out]
  n412 = call "ONL.vi"() -> ()  [unwired: 5 in, 15 out]
  n413 = call "ONL_Query.vi"() -> ()  [unwired: 4 in, 16 out]
  n414 = call "OpenStageEditorDialog.vi"() -> ()  [unwired: 3 in, 17 out]
  n415 = call "OVL.vi"() -> ()  [unwired: 5 in, 15 out]
  n416 = call "OVL_Query.vi"() -> ()  [unwired: 4 in, 16 out]
  n417 = call "POS.vi"() -> ()  [unwired: 5 in, 15 out]
  n418 = call "RBT.vi"() -> ()  [unwired: 2 in, 18 out]
  n419 = call-poly "REC.vi"() -> ()  [unwired: 19 in, 1 out]
  n420 = call "REL.vi"() -> ()  [unwired: 4 in, 16 out]
  n421 = call "REL_Query.vi"() -> ()  [unwired: 5 in, 15 out]
  n422 = call "RPA.vi"() -> ()  [unwired: 6 in, 14 out]
  n423 = call "RST.vi"() -> ()  [unwired: 5 in, 15 out]
  n424 = call "RTR.vi"() -> ()  [unwired: 3 in, 17 out]
  n425 = call "RTR_Query.vi"() -> ()  [unwired: 2 in, 18 out]
  n426 = call "SAI.vi"() -> ()  [unwired: 4 in, 16 out]
  n427 = call "MOD.vi"() -> ()  [unwired: 5 in, 15 out]
  n428 = call "MOD_Query.vi"() -> ()  [unwired: 5 in, 15 out]
  n429 = call "REC RATE.vi"() -> ()  [unwired: 19 in, 1 out]
  n430 = call "REC START.vi"() -> ()  [unwired: 19 in, 1 out]
  n431 = call "REC STOP.vi"() -> ()  [unwired: 19 in, 1 out]
  n432 = call "REC TRACE.vi"() -> ()  [unwired: 19 in, 1 out]
  n433 = call "REC TRG.vi"() -> ()  [unwired: 19 in, 1 out]
  n434 = call-poly "REC_Query.vi"() -> ()  [unwired: 18 in, 2 out]
  n435 = call "SAM.vi"() -> ()  [unwired: 19 in, 1 out]
  n436 = call "SAM_Query.vi"() -> ()  [unwired: 18 in, 2 out]
  n437 = call "SAV.vi"() -> ()  [unwired: 5 in, 15 out]
  n438 = call "SCA.vi"() -> ()  [unwired: 4 in, 16 out]
  n439 = call "SCA_Query.vi"() -> ()  [unwired: 2 in, 18 out]
  n440 = call "SCH.vi"() -> ()  [unwired: 3 in, 17 out]
  n441 = call "SCH_Query.vi"() -> ()  [unwired: 2 in, 18 out]
  n442 = call "SCT.vi"() -> ()  [unwired: 3 in, 17 out]
  n443 = call "SCT_Query.vi"() -> ()  [unwired: 2 in, 18 out]
  n444 = call "SEP.vi"() -> ()  [unwired: 11 in, 9 out]
  n445 = call "SEP_Query.vi"() -> ()  [unwired: 7 in, 13 out]
  n446 = call "SMR_Query.vi"() -> ()  [unwired: 18 in, 2 out]
  n447 = call "SMV.vi"() -> ()  [unwired: 19 in, 1 out]
  n448 = call "SMV_Query.vi"() -> ()  [unwired: 18 in, 2 out]
  n449 = call "SPV.vi"() -> ()  [unwired: 19 in, 1 out]
  n450 = call "REC_Query DAT.vi"() -> ()  [unwired: 18 in, 2 out]
  n451 = call "REC_Query DAT to Array.vi"() -> ()  [unwired: 17 in, 3 out]
  n452 = call "REC_Query NUM.vi"() -> ()  [unwired: 18 in, 2 out]
  n453 = call "REC_Query RATE.vi"() -> ()  [unwired: 18 in, 2 out]
  n454 = call "REC_Query STATE.vi"() -> ()  [unwired: 18 in, 2 out]
  n455 = call "REC_Query TRACE.vi"() -> ()  [unwired: 18 in, 2 out]
  n456 = call "REC_Query TRG.vi"() -> ()  [unwired: 18 in, 2 out]
  n457 = call "SPV_Query.vi"() -> ()  [unwired: 18 in, 2 out]
  n458 = call "CPA.vi"() -> ()  [unwired: 19 in, 1 out]
  n459 = call "SMA.vi"() -> ()  [unwired: 4 in, 16 out]
  n460 = call "SMA_Query.vi"() -> ()  [unwired: 3 in, 17 out]
  n461 = call "SMO.vi"() -> ()  [unwired: 4 in, 16 out]
  n462 = call "SMO_Query.vi"() -> ()  [unwired: 5 in, 15 out]
  n463 = call "SPI.vi"() -> ()  [unwired: 3 in, 17 out]
  n464 = call "SPI_Query.vi"() -> ()  [unwired: 2 in, 18 out]
  n465 = call "SRA.vi"() -> ()  [unwired: 5 in, 15 out]
  n466 = call "SRA_Query.vi"() -> ()  [unwired: 5 in, 15 out]
  n467 = call "SRG.vi"() -> ()  [unwired: 6 in, 14 out]
  n468 = call "SRG_Query.vi"() -> ()  [unwired: 5 in, 15 out]
  n469 = call "SSA.vi"() -> ()  [unwired: 5 in, 15 out]
  n470 = call "SSA_Query.vi"() -> ()  [unwired: 5 in, 15 out]
  n471 = call "SSN_Query.vi"() -> ()  [unwired: 4 in, 16 out]
  n472 = call "SST.vi"() -> ()  [unwired: 5 in, 15 out]
  n473 = call "SST_Query.vi"() -> ()  [unwired: 5 in, 15 out]
  n474 = call "STA_Query.vi"() -> ()  [unwired: 5 in, 15 out]
  n475 = call "STE.vi"() -> ()  [unwired: 6 in, 14 out]
  n476 = call "STE_Query.vi"() -> ()  [unwired: 6 in, 14 out]
  n477 = call "TCT_Query.vi"() -> ()  [unwired: 2 in, 18 out]
  n478 = call "TCV_Query.vi"() -> ()  [unwired: 5 in, 15 out]
  n479 = call "TIM.vi"() -> ()  [unwired: 5 in, 15 out]
  n480 = call "TIM_Query.vi"() -> ()  [unwired: 2 in, 18 out]
  n481 = call "TIO_Query.vi"() -> ()  [unwired: 2 in, 18 out]
  n482 = call "TMC_Query.vi"() -> ()  [unwired: 2 in, 18 out]
  n483 = call "TMP_Query.vi"() -> ()  [unwired: 2 in, 18 out]
  n484 = call "TNC_Query.vi"() -> ()  [unwired: 2 in, 18 out]
  n485 = call "TNR_Query.vi"() -> ()  [unwired: 2 in, 18 out]
  n486 = call "TPC_Query.vi"() -> ()  [unwired: 2 in, 18 out]
  n487 = call "TRC_Query.vi"() -> ()  [unwired: 2 in, 18 out]
  n488 = call "TRO.vi"() -> ()  [unwired: 4 in, 16 out]
  n489 = call "TRO_Query.vi"() -> ()  [unwired: 4 in, 16 out]
  n490 = call "TVI_Query.vi"() -> ()  [unwired: 3 in, 17 out]
  n491 = call "UCL.vi"() -> ()  [unwired: 19 in, 1 out]
  n492 = call "UCL_Query.vi"() -> ()  [unwired: 18 in, 2 out]
  n493 = call "VLS_Query.vi"() -> ()  [unwired: 2 in, 18 out]
  n494 = call "VST_Query.vi"() -> ()  [unwired: 2 in, 18 out]
  n495 = call "WAA.vi"() -> ()  [unwired: 4 in, 16 out]
  n496 = call "WPA.vi"() -> ()  [unwired: 7 in, 13 out]
  n497 = call "TRI.vi"() -> ()  [unwired: 4 in, 16 out]
  n498 = call "TRI_Query.vi"() -> ()  [unwired: 4 in, 16 out]
  n499 = call "VLS.vi"() -> ()  [unwired: 4 in, 16 out]
  n500 = call "#9.vi"() -> ()  [unwired: 2 in, 18 out]
  n501 = call "DDL.vi"() -> ()  [unwired: 6 in, 14 out]
  n502 = call "DDL?.vi"() -> ()  [unwired: 5 in, 15 out]
  n503 = call "DTL?.vi"() -> ()  [unwired: 4 in, 16 out]
  n504 = call "GWD?.vi"() -> ()  [unwired: 6 in, 14 out]
  n505 = call "Send WG commands and wait for answers.vi"() -> ()  [unwired: 3 in, 17 out]
  n506 = call "SWT.vi"() -> ()  [unwired: 6 in, 14 out]
  n507 = call "SWT?.vi"() -> ()  [unwired: 4 in, 16 out]
  n508 = call "TGA.vi"() -> ()  [unwired: 5 in, 15 out]
  n509 = call "TGC.vi"() -> ()  [unwired: 3 in, 17 out]
  n510 = call "TGF.vi"() -> ()  [unwired: 3 in, 17 out]
  n511 = call "TGL?.vi"() -> ()  [unwired: 4 in, 16 out]
  n512 = call "TGS.vi"() -> ()  [unwired: 4 in, 16 out]
  n513 = call "TGT.vi"() -> ()  [unwired: 3 in, 17 out]
  n514 = call "TGT?.vi"() -> ()  [unwired: 2 in, 18 out]
  n515 = call "TLT?.vi"() -> ()  [unwired: 2 in, 18 out]
  n516 = call "TWC.vi"() -> ()  [unwired: 2 in, 18 out]
  n517 = call "TWG?.vi"() -> ()  [unwired: 2 in, 18 out]
  n518 = call "TWS.vi"() -> ()  [unwired: 5 in, 15 out]
  n519 = call "TWS?.vi"() -> ()  [unwired: 7 in, 13 out]
  n520 = call "WAV CFG.vi"() -> ()  [unwired: 5 in, 15 out]
  n521 = call "WAV.vi"() -> ()  [unwired: 20 in, 8 out]
  n522 = call "WAV?.vi"() -> ()  [unwired: 4 in, 16 out]
  n523 = call "WCL.vi"() -> ()  [unwired: 5 in, 15 out]
  n524 = call "WGC.vi"() -> ()  [unwired: 4 in, 16 out]
  n525 = call "WGC?.vi"() -> ()  [unwired: 5 in, 15 out]
  n526 = call "WGO.vi"() -> ()  [unwired: 4 in, 16 out]
  n527 = call "WGO?.vi"() -> ()  [unwired: 5 in, 15 out]
  n528 = call "WGR.vi"() -> ()  [unwired: 2 in, 18 out]
  n529 = call "WMS.vi"() -> ()  [unwired: 5 in, 15 out]
  n530 = call "WMS?.vi"() -> ()  [unwired: 5 in, 15 out]
  n531 = call "WOS.vi"() -> ()  [unwired: 5 in, 15 out]
  n532 = call "WOS?.vi"() -> ()  [unwired: 4 in, 16 out]
  n533 = call "WSL.vi"() -> ()  [unwired: 4 in, 16 out]
  n534 = call "WSL?.vi"() -> ()  [unwired: 4 in, 16 out]
  n535 = call "WTO.vi"() -> ()  [unwired: 6 in, 14 out]
  n536 = call "WTR.vi"() -> ()  [unwired: 5 in, 15 out]
  n537 = call "WTR?.vi"() -> ()  [unwired: 4 in, 16 out]
  n538 = call "WGI?.vi"() -> ()  [unwired: 5 in, 15 out]
  n539 = call "WGN?.vi"() -> ()  [unwired: 5 in, 15 out]
  n540 = call "WGS?.vi"() -> ()  [unwired: 5 in, 15 out]
  n541 = call "ConvertStatusRegisterToAxisStatus.vi"() -> ()  [unwired: 18 in, 2 out]
  n542 = call "ConvertStatusRegisterToSystemStatus.vi"() -> ()  [unwired: 18 in, 2 out]
  n543 = call "ConvertStatusRegistersToAxisStatusArray.vi"() -> ()  [unwired: 18 in, 2 out]
  n544 = call "ConvertStatusRegistersToSystemStatusArray.vi"() -> ()  [unwired: 18 in, 2 out]
  n545 = call "Analyse input string for terminal.vi"() -> ()  [unwired: 2 in, 18 out]
  n546 = call "Assign booleans from string to axes.vi"() -> ()  [unwired: 5 in, 15 out]
  n547 = call "Assign DRC values.vi"() -> ()  [unwired: 3 in, 17 out]
  n548 = call "Assign DRT values from string.vi"() -> ()  [unwired: 7 in, 13 out]
  n549 = call "Assign NaN for chosen axes.vi"() -> ()  [unwired: 4 in, 16 out]
  n550 = call "Assign SPA values from string to axes.vi"() -> ()  [unwired: 7 in, 13 out]
  n551 = call "Assign three values from string to axes.vi"() -> ()  [unwired: 3 in, 17 out]
  n552 = call "Assign values from string to axes.vi"() -> ()  [unwired: 6 in, 14 out]
  n553 = call "Axes_settled.vi"() -> ()  [unwired: 5 in, 15 out]
  n554 = call "Boolean array calculations.vi"() -> ()  [unwired: 4 in, 16 out]
  n555 = call "Build channel query command substring.vi"() -> ()  [unwired: 7 in, 13 out]
  n556 = call "Build command substring.vi"() -> ()  [unwired: 7 in, 13 out]
  n557 = call "Build DIO_Query query command substring.vi"() -> ()  [unwired: 6 in, 14 out]
  n558 = call "Build MVS command substring.vi"() -> ()  [unwired: 6 in, 14 out]
  n559 = call "Build num command substring.vi"() -> ()  [unwired: 3 in, 17 out]
  n560 = call "Build query command substring.vi"() -> ()  [unwired: 5 in, 15 out]
  n561 = call "Build REL_Query query command substring.vi"() -> ()  [unwired: 5 in, 15 out]
  n562 = call "Build SPA command substring.vi"() -> ()  [unwired: 10 in, 10 out]
  n563 = call "Build SPA query command substring.vi"() -> ()  [unwired: 5 in, 15 out]
  n564 = call "Build stringplusnum substring.vi"() -> ()  [unwired: 10 in, 10 out]
  n565 = call "Build WAV command substring.vi"() -> ()  [unwired: 19 in, 9 out]
  n566 = call "Commanded axes connected_query.vi"() -> ()  [unwired: 3 in, 17 out]
  n567 = call "Commanded stage name available_Query.vi"() -> ()  [unwired: 3 in, 17 out]
  n568 = call "Convert error to warning.vi"() -> ()  [unwired: 2 in, 18 out]
  n569 = call "Convert num array to string.vi"() -> ()  [unwired: 2 in, 18 out]
  n570 = call "Convert num value to syntax selection.vi"() -> ()  [unwired: 1 in, 19 out]
  n571 = call "Count occurrences in string.vi"() -> ()  [unwired: 2 in, 18 out]
  n572 = call "Cut out additional spaces.vi"() -> ()  [unwired: 2 in, 18 out]
  n573 = call "Decode status bit.vi"() -> ()  [unwired: 2 in, 18 out]
  n574 = call "Define axes to command from boolean array.vi"() -> ()  [unwired: 4 in, 16 out]
  n575 = call "Define connected stages with dialog.vi"() -> ()  [unwired: 2 in, 18 out]
  n576 = call "Determine angular axis.vi"() -> ()  [unwired: 4 in, 16 out]
  n577 = call "GCSTranslateError.vi"() -> ()  [unwired: 1 in, 19 out]
  n578 = call "General wait for movement to stop.vi"() -> ()  [unwired: 8 in, 12 out]
  n579 = call "Get all axes.vi"() -> ()  [unwired: 1 in, 19 out]
  n580 = call "Get arrays without blanks.vi"() -> ()  [unwired: 3 in, 17 out]
  n581 = call "Get Controller Name from IDN.vi"() -> ()  [unwired: 2 in, 18 out]
  n582 = call "Get lines and values from string.vi"() -> ()  [unwired: 2 in, 18 out]
  n583 = call "Get lines from string.vi"() -> ()  [unwired: 3 in, 17 out]
  n584 = call "Split text segments from line.vi"() -> ()  [unwired: 19 in, 1 out]
  n585 = call "Get Slave Device Info.vi"() -> ()  [unwired: 2 in, 18 out]
  n586 = call "GCS3_Prepare_Motion_Error.vi"() -> ()  [unwired: 17 in, 3 out]
  n587 = call-poly "ConvertStatusRegister.vi"() -> ()  [unwired: 18 in, 2 out]
  n588 = call "Assign two values from string to axes.vi"() -> ()  [unwired: 3 in, 17 out]
  n589 = call "Build HIA command substring.vi"() -> ()  [unwired: 4 in, 16 out]
  n590 = call "Combine axes arrays.vi"() -> ()  [unwired: 2 in, 18 out]
  n591 = call "CST handler.vi"() -> ()  [unwired: 6 in, 14 out]
  n592 = call "Get string array size without blanks.vi"() -> ()  [unwired: 1 in, 19 out]
  n593 = call "Get total number of commanded axes.vi"() -> ()  [unwired: 2 in, 18 out]
  n594 = call "How often does string contain regular expression_Query.vi"() -> ()  [unwired: 2 in, 18 out]
  n595 = call "HasMotionError.vi"() -> ()  [unwired: 18 in, 2 out]
  n596 = call "Increase array size.vi"() -> ()  [unwired: 3 in, 17 out]
  n597 = call "InMotion.vi"() -> ()  [unwired: 17 in, 3 out]
  n598 = call "IsControllerBusy.vi"() -> ()  [unwired: 18 in, 2 out]
  n599 = call-poly "Is command present in HLP answer_Query.vi"() -> ()  [unwired: 5 in, 15 out]
  n600 = call "Longlasting one-axis command.vi"() -> ()  [unwired: 7 in, 13 out]
  n601 = call "Manual VMO.vi"() -> ()  [unwired: 6 in, 14 out]
  n602 = call "Move axes to their middle position.vi"() -> ()  [unwired: 5 in, 15 out]
  n603 = call "Multi Axis Query.vi"() -> ()  [unwired: 14 in, 2 out]
  n604 = call "Parse KLS_Query type answer by type.vi"() -> ()  [unwired: 3 in, 17 out]
  n605 = call "Parse qLOG Answer.vi"() -> ()  [unwired: 18 in, 2 out]
  n606 = call "Parse qUSG CMD Answer.vi"() -> ()  [unwired: 18 in, 2 out]
  n607 = call "Parse qUSG PAM Answer.vi"() -> ()  [unwired: 18 in, 2 out]
  n608 = call "Parse qUSG SYS Answer.vi"() -> ()  [unwired: 18 in, 2 out]
  n609 = call "ReadControllerInformation.vi"() -> ()  [unwired: 15 in, 5 out]
  n610 = call "Return single characters from string.vi"() -> ()  [unwired: 3 in, 17 out]
  n611 = call "Return space.vi"() -> ()  [unwired: 2 in, 18 out]
  n612 = call "Round with options.vi"() -> ()  [unwired: 4 in, 16 out]
  n613 = call "Select axis.vi"() -> ()  [unwired: 2 in, 18 out]
  n614 = call "Select values for chosen axes.vi"() -> ()  [unwired: 5 in, 15 out]
  n615 = call "Select with boolean array input.vi"() -> ()  [unwired: 4 in, 16 out]
  n616 = call "Selection to String array.vi"() -> ()  [unwired: 2 in, 18 out]
  n617 = call "Send string and wait for answer or timeout.vi"() -> ()  [unwired: 6 in, 14 out]
  n618 = call "Set RON and return RON status.vi"() -> ()  [unwired: 5 in, 15 out]
  n619 = call "Split multiple axes command.vi"() -> ()  [unwired: 9 in, 11 out]
  n620 = call "String with ASCII code conversion.vi"() -> ()  [unwired: 1 in, 19 out]
  n621 = call "Substract axes array subset from axes array.vi"() -> ()  [unwired: 2 in, 18 out]
  n622 = call "Unbunde/bundle interface clusters for PI Terminal.vi"() -> ()  [unwired: 6 in, 14 out]
  n623 = call "Wait for answer 0 or 1 without polling.vi"() -> ()  [unwired: 5 in, 15 out]
  n624 = call "Wait for answer of longlasting command.vi"() -> ()  [unwired: 3 in, 17 out]
  n625 = call "Wait for axes to stop.vi"() -> ()  [unwired: 7 in, 13 out]
  n626 = call "Wait for controller ready.vi"() -> ()  [unwired: 4 in, 16 out]
  n627 = call "GCSArray_difference.vi"() -> ()  [unwired: 3 in, 17 out]
  n628 = call "GCSArray_header_read.vi"() -> ()  [unwired: 3 in, 17 out]
  n629 = call "GCSArray_import.vi"() -> ()  [unwired: 3 in, 17 out]
  n630 = call "GCSArray_intersection.vi"() -> ()  [unwired: 3 in, 17 out]
  n631 = call "GCSArray_regex_matches.vi"() -> ()  [unwired: 4 in, 16 out]
  n632 = call "GCSArray_regex_select.vi"() -> ()  [unwired: 4 in, 16 out]
  n633 = call "GCSArray_regex_string.vi"() -> ()  [unwired: 2 in, 18 out]
  n634 = call "GCSArray_valid.vi"() -> ()  [unwired: 4 in, 16 out]
  n635 = call "Parse_FRH_Type_String.vi"() -> ()  [unwired: 3 in, 17 out]
  n636 = call "Sep axes ini result in order.vi"() -> ()  [unwired: 2 in, 18 out]
  n637 = call "StopAllMotion.vi"() -> ()  [unwired: 19 in, 1 out]
  n638 = call "C413_Configuration_Setup.vi"() -> ()  [unwired: 14 in, 6 out]
  n639 = call "C702_Configuration_Setup.vi"() -> ()  [unwired: 14 in, 6 out]
  n640 = call "C843_Configuration_Setup.vi"() -> ()  [unwired: 15 in, 5 out]
  n641 = call "C843_PM_Configuration_Setup.vi"() -> ()  [unwired: 15 in, 5 out]
  n642 = call "C866_Configuration_Setup.vi"() -> ()  [unwired: 13 in, 7 out]
  n643 = call "C867_Configuration_Setup.vi"() -> ()  [unwired: 12 in, 8 out]
  n644 = call "C867_Configuration_Setup_Rev2.vi"() -> ()  [unwired: 11 in, 9 out]
  n645 = call "C867_Multiaxis_Configuration_Setup.vi"() -> ()  [unwired: 13 in, 7 out]
  n646 = call "C877_Configuration_Setup.vi"() -> ()  [unwired: 11 in, 9 out]
  n647 = call "C884_Configuration_Setup.vi"() -> ()  [unwired: 12 in, 8 out]
  n648 = call "C885_Configuration_Setup.vi"() -> ()  [unwired: 10 in, 10 out]
  n649 = call "C885_SlaveDevice_Configuration_Setup.vi"() -> ()  [unwired: 6 in, 14 out]
  n650 = call "C886_Configuration_Setup.vi"() -> ()  [unwired: 7 in, 13 out]
  n651 = call "C887_Configuration_Setup.vi"() -> ()  [unwired: 13 in, 7 out]
  n652 = call "C891_Configuration_Setup.vi"() -> ()  [unwired: 12 in, 8 out]
  n653 = call "E135_Configuration_Setup.vi"() -> ()  [unwired: 4 in, 16 out]
  n654 = call "E516_Configuration_Setup.vi"() -> ()  [unwired: 11 in, 9 out]
  n655 = call "E517_Configuration_Setup.vi"() -> ()  [unwired: 13 in, 7 out]
  n656 = call "E518_Configuration_Setup.vi"() -> ()  [unwired: 12 in, 8 out]
  n657 = call "E709_Configuration_Setup.vi"() -> ()  [unwired: 14 in, 6 out]
  n658 = call "E710_Configuration_Setup.vi"() -> ()  [unwired: 12 in, 8 out]
  n659 = call "E712_Configuration_Setup.vi"() -> ()  [unwired: 15 in, 5 out]
  n660 = call "E725_Configuration_Setup.vi"() -> ()  [unwired: 14 in, 6 out]
  n661 = call "E727_Configuration_Setup.vi"() -> ()  [unwired: 14 in, 6 out]
  n662 = call "E753_Configuration_Setup.vi"() -> ()  [unwired: 13 in, 7 out]
  n663 = call "E754_Configuration_Setup.vi"() -> ()  [unwired: 13 in, 7 out]
  n664 = call "E755_Configuration_Setup.vi"() -> ()  [unwired: 12 in, 8 out]
  n665 = call "E761_Configuration_Setup.vi"() -> ()  [unwired: 11 in, 9 out]
  n666 = call "E816_Configuration_Setup.vi"() -> ()  [unwired: 10 in, 10 out]
  n667 = call "E861_Configuration_Setup.vi"() -> ()  [unwired: 12 in, 8 out]
  n668 = call "E870_Configuration_Setup.vi"() -> ()  [unwired: 6 in, 14 out]
  n669 = call "E871_Configuration_Setup.vi"() -> ()  [unwired: 12 in, 8 out]
  n670 = call "E871_Configuration_Setup_Rev2.vi"() -> ()  [unwired: 7 in, 13 out]
  n671 = call "E872_Configuration_Setup.vi"() -> ()  [unwired: 6 in, 14 out]
  n672 = call "E873_Configuration_Setup.vi"() -> ()  [unwired: 11 in, 9 out]
  n673 = call "E874_Configuration_Setup.vi"() -> ()  [unwired: 10 in, 10 out]
  n674 = call "F206_Configuration_Setup.vi"() -> ()  [unwired: 13 in, 7 out]
  n675 = call "HydraPollux_Configuration_Setup.vi"() -> ()  [unwired: 13 in, 7 out]
  n676 = call "M8X0_Configuration_Setup.vi"() -> ()  [unwired: 13 in, 7 out]
  n677 = call "Mercury_Configuration_Setup.vi"() -> ()  [unwired: 14 in, 6 out]
  n678 = call "Mercury_GCS_Configuration_Setup.vi"() -> ()  [unwired: 13 in, 7 out]
  n679 = call "PI Terminal.vi"() -> ()  [unwired: 20 out]
